vi "NKTP_API_ReadRegisterU8_Example.vi"() -> ()   [LabVIEW 2011]
uses:
  <instrlib>/NKTP_API/NKTP_API.lvlib
panel:
  out "error out":errorcluster
  out "Value":u8 format="%.0x"
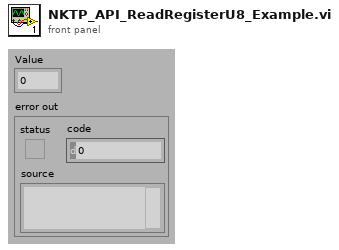
[diagram p1: front panel]
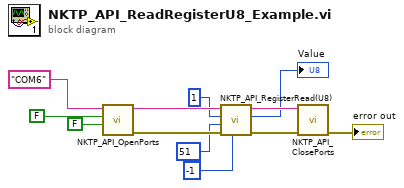
[diagram p0: block diagram]
diagram:
  n1 = call <instrlib>:"NKTP_API_OpenPorts.vi"("liveMode"=FALSE ("LiveMode"), "autoMode"=FALSE ("AutoMode"), "portnames"="COM6") -> ("error out"=w11:errorcluster, "portnames out"=w12:string)  [unwired: 7 in]
  n2 = call <instrlib>:"NKTP_API_RegisterRead(U8).vi"("index"=i16 -1 ("Index"), "error in"=w11, "regId"=u8 51 ("RegId"), "devId"=u8 1 ("DevId"), "portname"=w12) -> ("error out"=w7:errorcluster, "value"=→"Value":u8, "portname out"=w8:string)  [unwired: 4 in]
  n3 = call <instrlib>:"NKTP_API_ClosePorts.vi"("error in"=w7, "portnames"=w8) -> ("error out"=→"error out":errorcluster)  [unwired: 8 in, 1 out]
